vi "TCP 1.vi"() -> ()   [LabVIEW 2023]
uses:
  <vilib>/picture/picture.llb/Draw True-Color Pixmap.vi
panel:
  in  "Screen On/Off":bool
  out "Drone Camera":picture
  in  "Stop Dashboard":bool
  out "error out":errorcluster
  out "data out":string
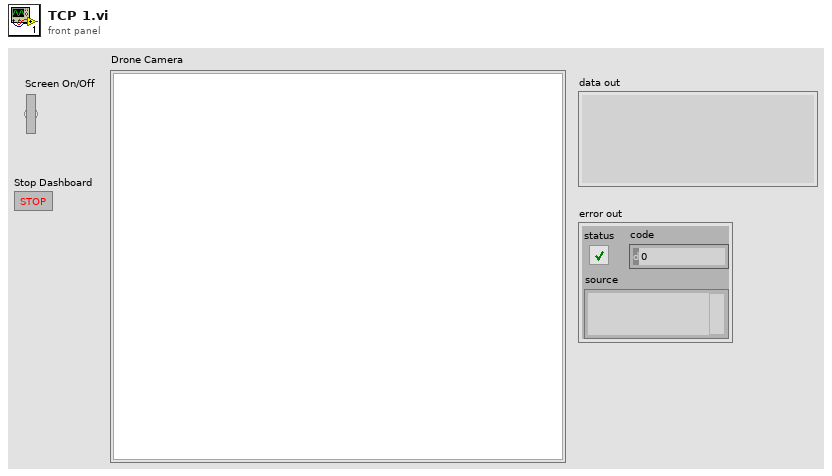
[diagram p1: front panel]
types:
  T1 = enum16{"Standard", "Buffered", "CRLF", "Immediate"}
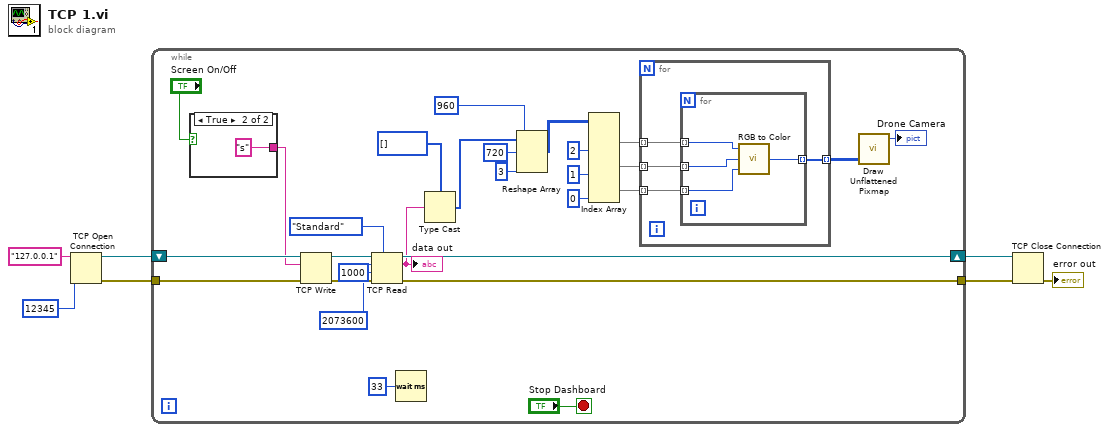
[diagram p0: block diagram]
diagram:
  n1 = TCP Open Connection(address="127.0.0.1", remote port or service name=u16 12345) -> (connection ID=w7:refnum<k5>, error out=w3:errorcluster)  [unwired: 3 in]
  n2 = while {
    shift-right: [w33] -> w6
    shift-left: w7 -> [w35]
    tunnel: w3 -> [w32]
    tunnel: [w30] -> w2
    stop <- "Stop Dashboard" stop-if-true
    n3 = case shown="True" "Screen On/Off" {
      tunnel: [_ "s"] -> w9
      frame False {
      }
      frame True {
      }
    }
    n4 = TCP Write(connection ID=w35, data in=w9, error in (no error)=w32) -> (connection ID out=w34:refnum<k5>, error out=w31:errorcluster)  [unwired: 1 in, 1 out]
    n5 = TCP Read(connection ID=w34, bytes to read=2073600, error in (no error)=w31, 7:T1."Standard" ("mode (standard)"), 9:1000 ("timeout ms (25000)")) -> (connection ID out=w33:refnum<k5>, data out=w24:string, error out=w30:errorcluster)
    "data out" <- w24
    n6 = Wait (ms)(milliseconds to wait=u32 33) -> ()  [unwired: 1 out]
    n7 = Type Cast(type=u8[] [], x=w24) -> (*(type *) &x=w22:u8[])
    n8 = Reshape Array(w22, 720 ("dimension size"), 960 ("dimension size"), 3 ("dimension size")) -> (w18:u8[][][])
    n9 = Index Array(array=w18, index (dim 2) #1=2 ("disabled index (col)"), index (dim 2) #2=1 ("index (col)"), index (dim 2) #3=0 ("index (col)")) -> (element #1=w14:u8[][], element #2=w13:u8[][], element #3=w12:u8[][])  [unwired: 6 in]
    n10 = for {
      tunnel: w14 -> [w40] mode=indexing
      tunnel: w13 -> [w39] mode=indexing
      tunnel: w12 -> [w38] mode=indexing
      tunnel: [w37] -> w11 mode=indexing
      n11 = for {
        tunnel: w40 -> [w44] mode=indexing
        tunnel: w39 -> [w43] mode=indexing
        tunnel: w38 -> [w42] mode=indexing
        tunnel: [w41] -> w37 mode=indexing
        n12 = call <vilib>:"RGB to Color.vi"("B"=w42, "G"=w43, "R"=w44) -> ("Color"=w41:u32)
      }
    }
    n13 = call-poly <vilib>:"Draw Unflattened Pixmap.vi"("data (RGB format)"=w11) -> ("new picture"=→"Drone Camera":picture)  [unwired: 8 in]
  }
  n14 = TCP Close Connection(connection ID=w6, error in (no error)=w2) -> (error out=→"error out":errorcluster)  [unwired: 1 in, 1 out]
